vi "Init.vi"(8 "error in (no error)":errorcluster, 11 "Input Name":string) -> (0 "error out":errorcluster, 3 "GetInputMute out":refnum<class "GetInputMute.lvclass">)   [LabVIEW 2022 SP3, in "obs-websocket-lv.lvlib" / "GetInputMute.lvclass"]
uses:
  GetInputMute.lvclass
  GetInputMute.lvclass/GetInputMute.ctl
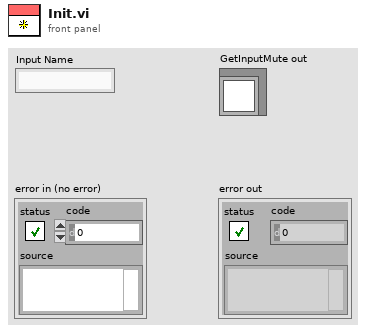
[diagram p1: front panel]
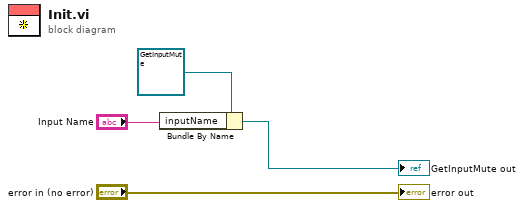
[diagram p0: block diagram]
diagram:
  n1 = Bundle By Name(cluster=refnum<class "GetInputMute.lvclass"> refnum ("GetInputMute in"), "inputName"="Input Name") -> (→"GetInputMute out":refnum<class "GetInputMute.lvclass">)
  "error out" <- "error in (no error)"
